vi "Delay.vi"(0 "initial value":dbl, 1 "stream in":T1) -> (2 "stream out":T1)   [LabVIEW 2023]
uses:
  <extravilib>/ChannelInstances/Stream-dbl/)Channel.ctl
  <extravilib>/ChannelInstances/Stream-dbl/Read With Abort.vi
  <extravilib>/ChannelInstances/Stream-dbl/Write With Abort.vi
  <extravilib>/ChannelInstances/Stream-dbl/EndpointRead.vi
  <extravilib>/ChannelInstances/Stream-dbl/Endpoint.vi
  <extravilib>/ChannelInstances/Stream-dbl/)Channel.vi
  <resource>/ChannelSupport/_ChannelSupport/WaitIfNeeded.vi
  <extravilib>/ChannelInstances/Stream-dbl.lvlib
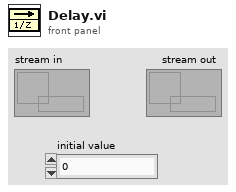
[diagram p1: front panel]
types:
  T1 = typedef "Stream-dbl.lvlib/)Channel.ctl" = refnum<queue>
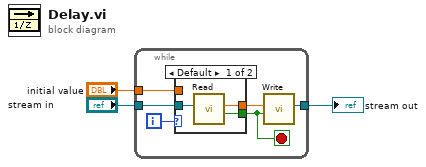
[diagram p0: block diagram]
diagram:
  n1 = while {
    tunnel: [w5] -> w1
    tunnel: "stream in" -> [w9]
    tunnel: "initial value" -> [w8]
    i -> [w7]
    stop <- w4 stop-if-true
    n2 = case shown="Default" w7 {
      tunnel: w9 -> [w12 _]
      tunnel: w8 -> [_ w13]
      tunnel: [w11 w13] -> w6
      tunnel: [w10 _] -> w4
      frame Default {
        n3 = call <extravilib>:"Read.vi"("channel"=w12) -> ("last element?"=w10:bool, "element"=w11:dbl)  [unwired: 6 in, 3 out]
      }
      frame 0 {
      }
    }
    n4 = call <extravilib>:"Write.vi"("last element? (F)"=w4, "element"=w6) -> ("channel"=w5:T1)  [unwired: 7 in, 2 out]
  }
  "stream out" <- w1
